vi "Close VI Ref.vi"(8 "error in (no error)":errorcluster, 11 "LUnit Test Case In":refnum<class "LUnit Inheriting Test Case.lvclass">) -> (0 "error out":errorcluster, 3 "LUnit Test Case Out":refnum<class "LUnit Inheriting Test Case.lvclass">)   [LabVIEW 2020]
uses:
  LUnit Inheriting Test Case.lvclass
  C:/git/astemes-lunit/source/API/LUnit Test Case/LUnit Test Case.lvclass
  C:/git/astemes-lunit/source/Core/Runnable/Runnable.lvclass
  C:/git/astemes-lunit/source/API/LUnit Inheriting Test Case/LUnit Test Case/LUnit Inheriting Test Case.lvclass
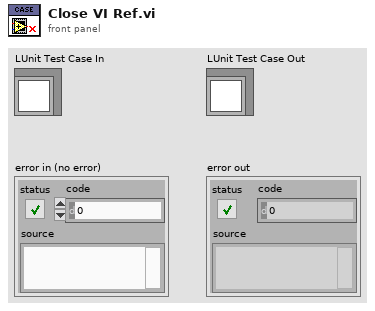
[diagram p1: front panel]
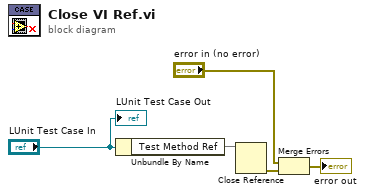
[diagram p0: block diagram]
diagram:
  n1 = Unbundle By Name("LUnit Test Case In") -> ("Test Method Ref"=w4)
  n2 = Close Reference(reference=w4) -> (error out=w5:errorcluster)  [unwired: 1 in]
  n3 = Merge Errors("error in (no error)", w5) -> (→"error out":errorcluster)
  "LUnit Test Case Out" <- "LUnit Test Case In"
